vi "TMP007 Example.vi"() -> ()   [LabVIEW 2014]
uses:
  <vilib>/myRIO/Instrument Drivers/Onboard IO/DIO/typedefs/DIO Reference.ctl
  <vilib>/myRIO/Common/Instrument Driver Framework/Utilities/typedefs/myRIO Generic Hardware Reference.ctl
  <vilib>/myRIO/Common/Instrument Driver Framework/Utilities/typedefs/Hardware Version Enum.ctl
  <vilib>/myRIO/Common/Instrument Driver Framework/Utilities/typedefs/myRIO v1.0 Reference.ctl
  <vilib>/myRIO/Common/Instrument Driver Framework/Utilities/typedefs/Generic FPGA Reference.ctl
  <vilib>/myRIO/Common/Instrument Driver Framework/myRIO v1.0/DIO/typedefs/DIO Channels List.ctl
  <vilib>/myRIO/Common/Instrument Driver Framework/myRIO v1.0/DIO/typedefs/DIO Channels Enum.ctl
  <vilib>/userdefined/High Color/nirio_resource_hc.ctl
  <vilib>/myRIO/Common/Instrument Driver Framework/Utilities/vis/Is FPGA Ref Available.vi
  <vilib>/myRIO/Common/Instrument Driver Framework/myRIO v1.0/DIO/vis/myRIO v1.1 Open DIO.vi
  <vilib>/myRIO/Instrument Drivers/Onboard IO/DIO/vis/Write.vi
  <vilib>/myRIO/Common/Instrument Driver Framework/Utilities/vis/Validate Channels.vi
  <vilib>/myRIO/Common/Instrument Driver Framework/myRIO v1.0/DIO/vis/myRIO v1.0 Reserve DIO.vi
  <vilib>/myRIO/Common/Instrument Driver Framework/myRIO v1.0/Resource Manager/vis/myRIO v1.0 Reserve Channel List.vi
  <vilib>/myRIO/Common/Instrument Driver Framework/myRIO v1.0/DIO/vis/myRIO v1.0 Build MUX Configuration DIO.vi
  <vilib>/myRIO/Common/Instrument Driver Framework/myRIO v1.0/Resource Manager/vis/myRIO v1.0 Reserve Channel.vi
  <vilib>/myRIO/Common/Instrument Driver Framework/myRIO v1.0/Resource Manager/vis/myRIO v1.0 Unreserve Channel.vi
  <vilib>/myRIO/Common/Instrument Driver Framework/myRIO v1.0/Resource Manager/vis/myRIO v1.0 Create Configuration List.vi
  <vilib>/myRIO/Common/Instrument Driver Framework/myRIO v1.0/Resource Manager/vis/myRIO v1.0 Build Mutex Name.vi
  <vilib>/Utility/VariantDataType/GetNumericInfo.vi
  <vilib>/Utility/error.llb/Error Cluster From Error Code.vi
  <vilib>/myRIO/Common/Instrument Driver Framework/myRIO v1.0/myRIO v1.1 Open.vi
  <vilib>/myRIO/Common/Instrument Driver Framework/Utilities/vis/IO Manager.vi
  <vilib>/myRIO/Common/Instrument Driver Framework/Utilities/vis/Configuration Manager.vi
  <vilib>/myRIO/Common/Instrument Driver Framework/myRIO v1.0/Resource Manager/vis/myRIO v1.0 Configure IO.vi
  <vilib>/myRIO/Common/Instrument Driver Framework/myRIO v1.0/myRIO v1.0 Close.vi
  <vilib>/myRIO/Common/Instrument Driver Framework/myRIO v1.0/DIO/vis/myRIO v1.0 Write DIO.vi
  <vilib>/MakerHub/LINX/Public/Utilities/Open Local.vi
  <vilib>/myRIO/Express VI/Onboard IO/DO/DO Express VI.xnode
  <vilib>/myRIO/Instrument Drivers/Onboard IO/DIO/vis/myRIO DIO Open.xnode
  <vilib>/MakerHub/LINX/LMH-LINX.lvlib
  <vilib>/myRIO/Instrument Drivers/Onboard IO/DIO/DIO.lvlib
panel:
  out "Temp Readings":T1 {"Ambient Temp (°F)" format="%.2f °F"; "Ambient Temp (°C)" format="%.2f °C"; "Object Temp (°F)" format="%.2f °F"; "Object Temp (°C)" format="%.2f °C"}
  out "Conversion Time (S)":dbl format="%#_g s"
  in  "I2C Slave Address":u8=65 format="%x"
  in  "I2C Channel":u8=1
  out "Error Out":errorcluster
  out "Device Name":string
  out "ToF Loop Rate":u32
  in  "Wait (ms)":u32=10
  in  "Stop":bool
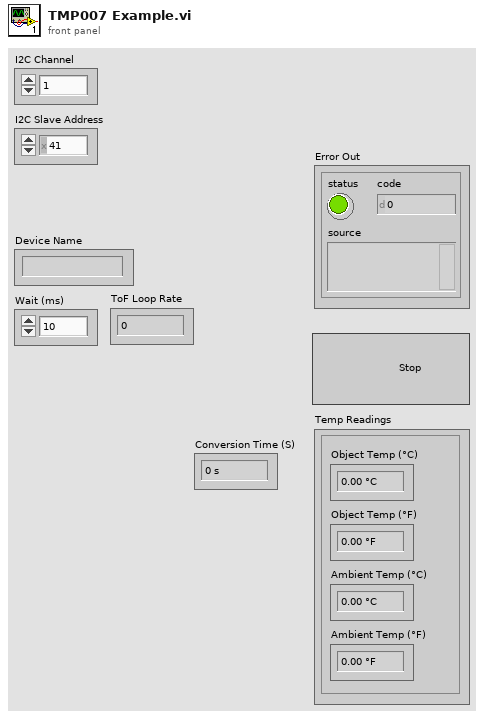
[diagram p1: front panel]
types:
  T1 = cluster{"Object Temp (°C)":dbl, "Object Temp (°F)":dbl, "Ambient Temp (°C)":dbl, "Ambient Temp (°F)":dbl}
  T2 = typedef "LMH-LINX.lvlib/LINX Ref.ctl" = cluster{"IO":T3, "Interface":T4, "LINX Device Config":T5}
  T3 = typedef "LMH-LINX.lvlib/Platform.ctl" = enum16{"Remote", "Local"}
  T4 = typedef "LMH-LINX.lvlib/Interface.ctl" = enum16{"Serial", "TCP"}
  T5 = typedef "LMH-LINX.lvlib/Device.lvlib/LINX Device Config.ctl" = cluster{"Interface":T4, "COM Port":refnum<visa-resource-name>, "TCP Configuration":T6, "Device Family":u8, "Device ID":u8, "Device Name":string, "TCP Ref":refnum<k5>, "Channels":T7}
  T6 = typedef "LMH-LINX.lvlib/Device.lvlib/TCP Config.ctl" = cluster{"IP Address":string, "Port":u16}
  T7 = typedef "LMH-LINX.lvlib/Channels.ctl" = cluster{"DI":u8[], "DO":u8[], "AI":u8[], "AO":u8[], "PWM":u8[], "QE":u8[], "UART":u8[], "I2C 2":u8[], "SPI":u8[], "CAN":u8[], "Servo":u8[], "AI Ref (V)":dbl, "AI Resolution (Bits)":u8, "AO Ref (V)":dbl, "AO Resolution (Bits)":u8}
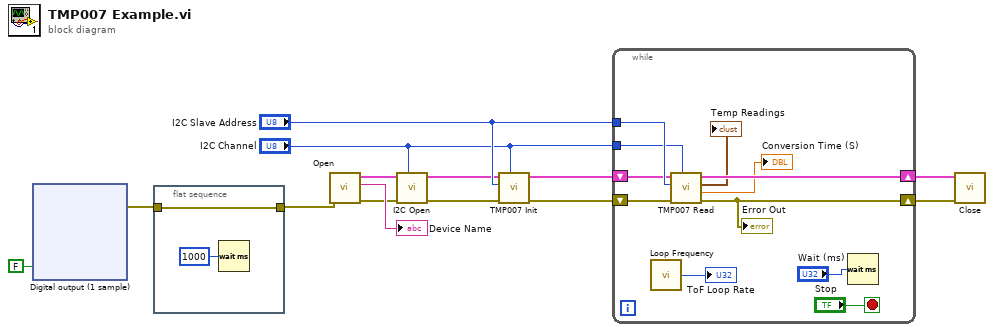
[diagram p0: block diagram]
diagram:
  n1 = xnode "Digital output (1 sample)"("Sensor Power (B/DIO7 (Pin 25))"=FALSE) -> ("error out"=w9:errorcluster)  [unwired: 1 in]
  n2 = flat-sequence {
    tunnel: w9 -> [w16]
    tunnel: [w16] -> w8
    frame #0 {
      n3 = Wait (ms)(milliseconds to wait=u32 1000) -> ()  [unwired: 1 out]
    }
  }
  n4 = call-poly <vilib>:"Open.vi"("Error In"=w8) -> ("Error Out"=w12:errorcluster, "Device Name"=→"Device Name":string, "LINX Resource"=w13:T2)  [unwired: 8 in]
  n5 = call <vilib>:"I2C Open.vi"("I2C Channel (0)"="I2C Channel", "Error In"=w12, "LINX Resource"=w13) -> ("Error Out"=w4:errorcluster, "LINX Resource"=w5:T2)  [unwired: 7 in]
  n6 = call "TMP007 Init.vi"("I2C Channel"="I2C Channel", "error in (no error)"=w4, "I2C Slave Address"="I2C Slave Address", "LINX Resource in"=w5) -> ("error out"=w3:errorcluster, "LINX Resource out"=w2:T2)  [unwired: 6 in]
  n7 = while {
    shift-right: [w20] -> w11
    shift-left: w2 -> [w23]
    shift-right: [w19] -> w10
    shift-left: w3 -> [w22]
    tunnel: "I2C Channel" -> [w24]
    tunnel: "I2C Slave Address" -> [w25]
    stop <- "Stop" stop-if-true
    n8 = call <vilib>:"Loop Frequency.vi"() -> ("Loop Rate (Hz)"=→"ToF Loop Rate":u32)
    n9 = call "TMP007 Read.vi"("I2C Channel"=w24, "error in (no error)"=w22, "I2C Slave Address"=w25, "LINX Resource in"=w23) -> ("error out"=w19:errorcluster, "Conversion Time (S)"=→"Conversion Time (S)":dbl, "Temp Readings"=→"Temp Readings":T1, "LINX Resource"=w20:T2)  [unwired: 4 in]
    "Error Out" <- w19
    n10 = Wait (ms)(milliseconds to wait="Wait (ms)") -> ()  [unwired: 1 out]
  }
  n11 = call <vilib>:"Close.vi"("Error In"=w10, "LINX Resource"=w11) -> ()  [unwired: 9 in, 1 out]
